vi "Filter Wheel Update Status.vi"(8 "error in (no error)":errorcluster, 11 "FW Status":T1={"State"=enum."Move Complete", "Positions"=[], "Names"=[], "Notch"=[], "Moving"=[FALSE, FALSE]}) -> (0 "error out":errorcluster)   [LabVIEW 2024]
uses:
  FW cluster Status.ctl
  FW enum status.ctl
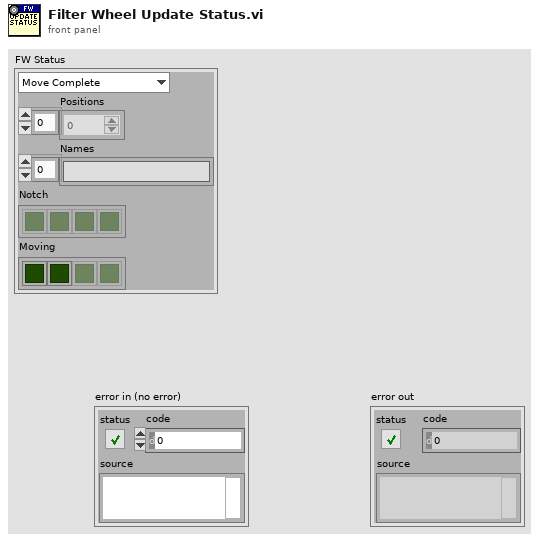
[diagram p1: front panel]
types:
  T1 = typedef "FW cluster Status.ctl" = cluster{"State":T2, "Positions":i32[], "Names":string[], "Notch":bool[], "Moving":bool[]}
  T2 = typedef "FW enum status.ctl" = enum16{"Initializing", "Moving", "Move Complete", "Error"}
  T3 = typedef "CC Current Status.ctl" = cluster{"Target":string, "Filter Position":string[]}
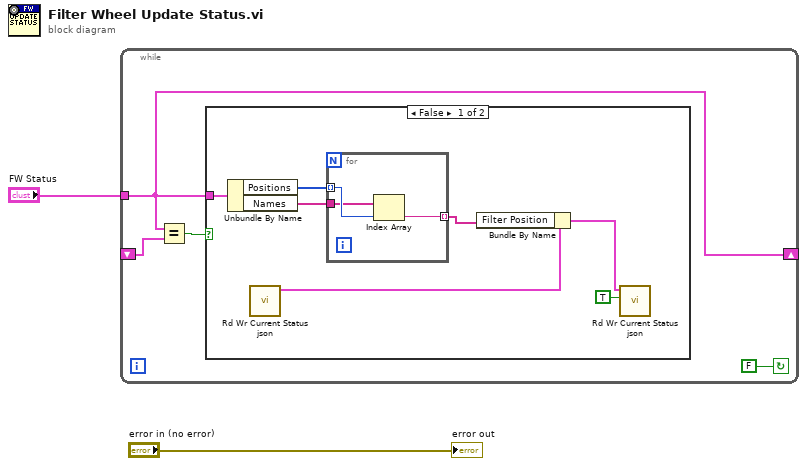
[diagram p0: block diagram]
diagram:
  n1 = while {
    tunnel: "FW Status" -> [w5]
    shift-right: [w5] -> _
    shift-left: _ -> [w4]
    stop <- FALSE continue-if-true
    n2 = Equal?(x=w5, y=w4) -> (x = y?=w3:bool)
    n3 = case shown="False" w3 {
      tunnel: w5 -> [w11 _]
      frame False {
        n4 = Unbundle By Name(w11) -> ("Positions"=w13:i32[], "Names"=w12:string[])
        n5 = call "Rd Wr Current Status json.vi"() -> ("Current Status"=w10:T3)  [unwired: 10 in, 1 out]
        n6 = for {
          tunnel: w13 -> [w16] mode=indexing
          tunnel: w12 -> [w15]
          tunnel: [w14] -> w7 mode=indexing
          n7 = Index Array(array=w15, index=w16) -> (element=w14:string)
        }
        n8 = Bundle By Name(cluster=w10, "Filter Position"=w7) -> (w9:T3)
        n9 = call "Rd Wr Current Status json.vi"("Write? (F:Read)"=TRUE, "Current Status"=w9) -> ()  [unwired: 8 in, 2 out]
      }
      frame True {
      }
    }
  }
  "error out" <- "error in (no error)"
